vi "Sheet Exists.vi"(8 "error in (no error)":errorcluster, 10 "Sheet Name":string, 11 "MS-Excel in":refnum<class "MS-Excel.lvclass">) -> (0 "error out":errorcluster, 2 "Exists":bool, 3 "MS-Excel out":refnum<class "MS-Excel.lvclass">)   [LabVIEW 2020, in "LabVIEW NPOI.lvlib" / "MS-Excel.lvclass"]
doc: "Checksif a sheet nammed <b>SheetName</b> exists in the associated workbook to the <b>Document</b>.\nReturn True if the sheet exists, false otherwise"
uses:
  MS-Excel.lvclass
  MS-Excel.lvclass/MS-Excel.ctl
  16bda17f-fd45-4b13-8a5f-fdac2f2a9084.vi
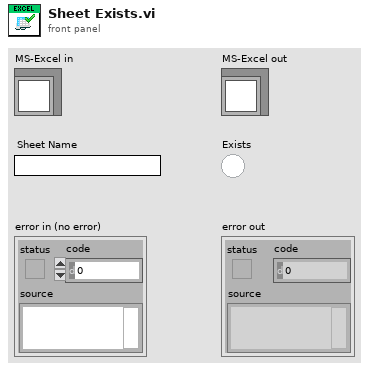
[diagram p1: front panel]
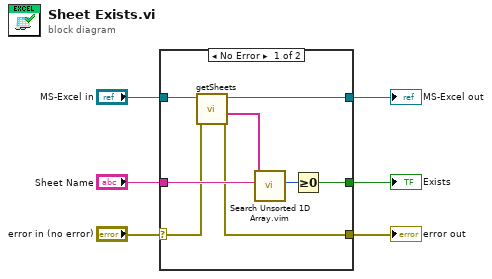
[diagram p0: block diagram]
diagram:
  n1 = case shown="No Error" "error in (no error)" {
    selector: "error in (no error)" -> [w10 w16]
    tunnel: [w9 w16] -> w5
    tunnel: [w13 w15] -> w3
    tunnel: "MS-Excel in" -> [w14 w15]
    tunnel: "Sheet Name" -> [w11 _]
    tunnel: [w7 _] -> w1
    frame No Error {
      n2 = call-dynamic "getSheets.vi"("error in (no error)"=w10, "MS-Excel in"=w14) -> ("error out"=w9:errorcluster, "Sheet Names"=w12:string[], "MS-Excel out"=w13:refnum<class "MS-Excel.lvclass">)  [unwired: 6 in, 1 out]
      n3 = call "Search Unsorted 1D Array.vim"("element"=w11, "unsorted 1D array"=w12) -> ("index of element"=w8:i32)  [unwired: 9 in]
      n4 = Greater Or Equal To 0?(x=w8) -> (x >= 0?=w7:bool)
    }
    frame Error {
    }
  }
  "error out" <- w5
  "MS-Excel out" <- w3
  "Exists" <- w1
